vi "SequenceEvent.ProgressChanged.vi"(4 "Progress":refnum<user-event>, 5 "Event Data":cluster{"sender":refnum<k24>, "e":refnum<k24>}, 6 "Control Ref":refnum<k24>, 7 "Event Common Data":T1) -> ()   [LabVIEW 2015, in "Simple Sequence Tools - Execution.lvlib"]
uses:
  Simple Sequence Tools - Execution.lvlib
  NationalInstruments.VeriStand.RealTimeSequenceDefinitionApi
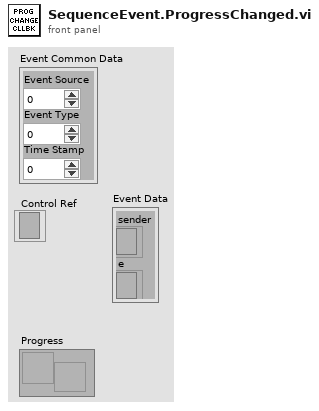
[diagram p1: front panel]
types:
  T1 = cluster{"Event Source":i32, "Event Type":u32, "Time Stamp":u32}
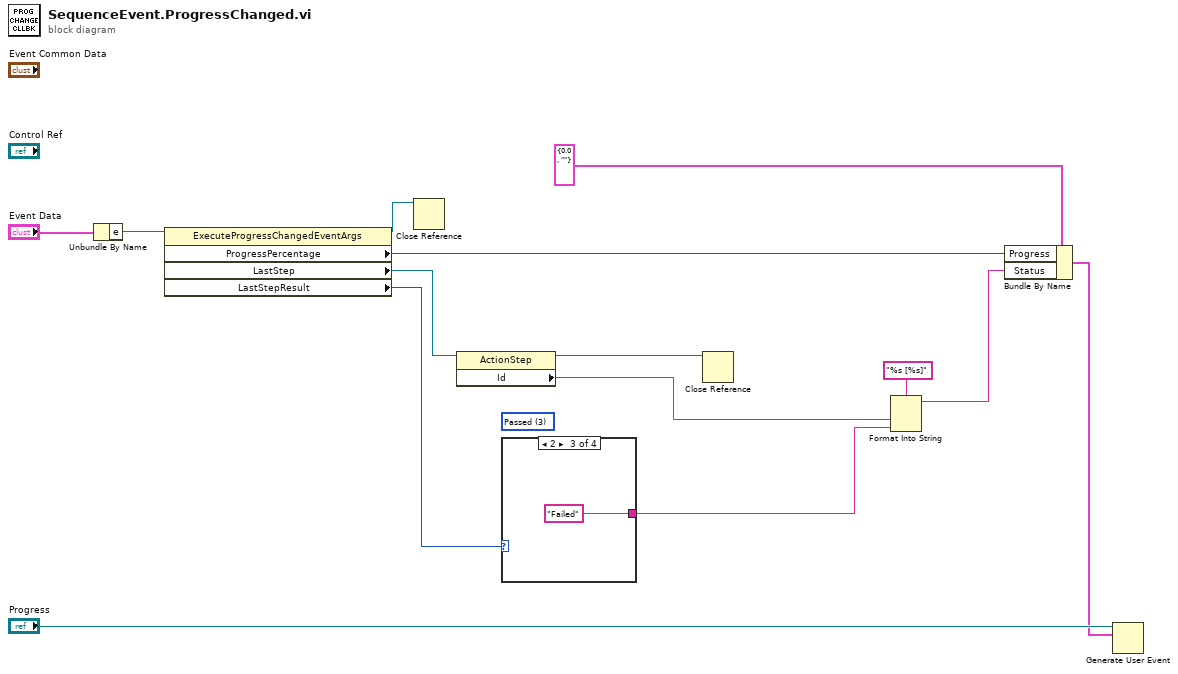
[diagram p0: block diagram]
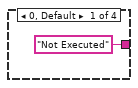
[diagram p2: hidden frame]
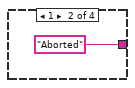
[diagram p3: hidden frame]
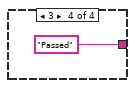
[diagram p4: hidden frame]
diagram:
  (unwired) 3 items=["NotExecuted", "Aborted", "Failed", "Passed"] ("LastStepResult")
  n1 = Unbundle By Name("Event Data") -> ("e"=w13:refnum<k24>)
  n2 = property class="ExecuteProgressChangedEventArgs"(reference=w13) -> (reference out=w4:refnum<k24>, "ProgressPercentage"=w9:i32, "LastStep"=w7:refnum<k24>, "LastStepResult"=w1:i32)  [unwired: 1 in, 1 out]
  n3 = Close Reference(reference=w4) -> ()  [unwired: 1 in, 1 out]
  n4 = property class="ActionStep"(reference=w7) -> (reference out=w5:refnum<k24>, "Id"=w6:string)  [unwired: 1 in, 1 out]
  n5 = case shown="2" w1 {
    tunnel: ["Not Executed" ("Status") "Aborted" ("Status") "Failed" ("Status") "Passed" ("Status")] -> w3
    frame 0, Default {
    }
    frame 1 {
    }
    frame 2 {
    }
    frame 3 {
    }
  }
  n6 = Close Reference(reference=w5) -> ()  [unwired: 1 in, 1 out]
  n7 = Format Into String(format string="%s [%s]", w6, w3) -> (resulting string=w2:string)  [unwired: 2 in, 1 out]
  n8 = Bundle By Name(cluster=cluster{"Progress":dbl, "Status":string} {"Progress"=0.0, "Status"=""} ("event data"), "Progress"=w9, "Status"=w2) -> (w10:cluster{"Progress":dbl, "Status":string})
  n9 = Generate User Event(user event="Progress", event data cluster=w10) -> ()  [unwired: 2 in, 2 out]
